vi "제목없음 3.vi"() -> ()   [LabVIEW 2017]
panel:
  out "부호없는 바이트 배열 2":u8[](array[numeric])
  out "Pack(4byte) 2":string
  in  "정수형 입력":i32=455000
  in  "소수형 입력":dbl=3.14 format="%#_13g"
  out "부호없는 바이트 배열":u8[](array[numeric])
  out "Pack(4byte)":string
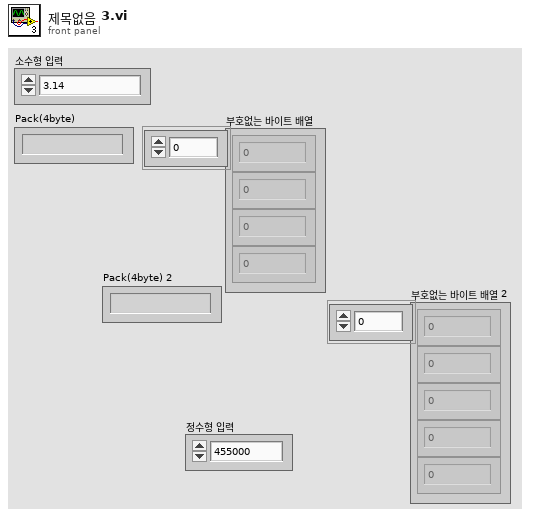
[diagram p1: front panel]
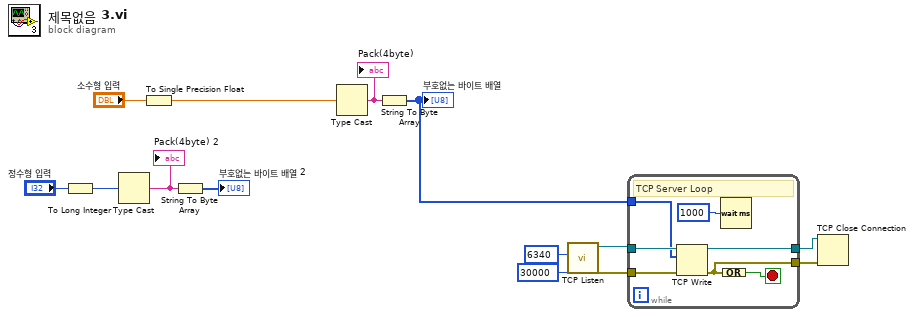
[diagram p0: block diagram]
diagram:
  n1 = To Long Integer(number="정수형 입력") -> (32bit integer=w3:i32)
  n2 = Type Cast(x=w3) -> (*(type *) &x=w4:string)  [unwired: 1 in]
  "Pack(4byte) 2" <- w4
  n3 = To Single Precision Float(number="소수형 입력") -> (single precision float=w11:sgl)
  n4 = String To Byte Array(string=w4) -> (unsigned byte array=→"부호없는 바이트 배열 2":u8[])
  n5 = Type Cast(x=w11) -> (*(type *) &x=w10:string)  [unwired: 1 in]
  "Pack(4byte)" <- w10
  n6 = String To Byte Array(string=w10) -> (unsigned byte array=w1:u8[])
  "부호없는 바이트 배열" <- w1
  n7 = call <vilib>:"TCP Listen.vi"("timeout ms (wait forever: -1)"=30000, "port"=u16 6340) -> ("error out"=w8:errorcluster, "connection ID"=w9:refnum<k5>)  [unwired: 5 in, 3 out]
  n8 = while {
    tunnel: w9 -> [w20]
    tunnel: w8 -> [w19]
    tunnel: [w18] -> w14
    tunnel: [w17] -> w13
    tunnel: w1 -> [w15]
    stop <- w16 stop-if-true
    # "TCP Server Loop"
    n9 = TCP Write(connection ID=w20, data in=w15, error in (no error)=w19) -> (connection ID out=w17:refnum<k5>, error out=w18:errorcluster)  [unwired: 2 out]
    n10 = Wait (ms)(milliseconds to wait=u32 1000) -> ()  [unwired: 1 out]
    n11 = Compound Arithmetic op=OR(w18) -> (w16:bool)
  }
  n12 = TCP Close Connection(connection ID=w13, error in (no error)=w14) -> ()  [unwired: 3 out]
